vi "Equi-Ripple BandPass.vi"   [LabVIEW 2020, in "NI_AALBase.lvlib"]
doc: "Generates a bandpass FIR filter with equi-ripple characteristics using the Parks-McClellan algorithm and the <B>higher pass freq</B>, <B>lower pass freq</B>, <B># of taps</B>, <B>lower stop freq</B>, <B>higher stop freq</B>, and <B>sampling freq: fs</B>. The Equi-Ripple BandPass VI then applies a linear-phase, bandpass filter to the input sequence <B>X</B> using the Convolution VI to obtain <B>Filtered X</B>. Wire data to the <B>X</B> input to determine the polymorphic instance to use or manually select the instance."
uses:
  <vilib>/Analysis/NI_AALBase.lvlib
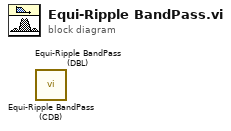
[diagram p0: block diagram]
diagram:
  n1 = call <vilib>:"Equi-Ripple BandPass (CDB).vi"() -> ()  [unwired: 8 in, 2 out]
  n2 = call <vilib>:"Equi-Ripple BandPass (DBL).vi"() -> ()  [unwired: 8 in, 2 out]
